vi "4 DDS.vi"(7 "clear DDS":bool, 8 "input valid":bool=TRUE, 9 "pdw in":T2 {"frequency shift" format="%#_12f"}, 10 "free DDS before me?":bool, 11 "new PDW in":bool) -> (0 "output valid":bool, 1 "state of every DDS":bool[](array[boolean]), 2 "have free DDS":bool, 3 "IQ out":T1)   [LabVIEW 2021]
doc: "transmit pulse with one free DDS inside.\nmust have no DDS before him (the distribute is to give the lowest mun DDS the pulse)"
uses:
  pulse_tx_vis/pdw.ctl
  pulse_tx_vis/CTL/mode_type.ctl
  <instrlib>/_niInstr/DSP/v1/Shared/Public/IQ Data.ctl
  <instrlib>/_niInstr/DSP/v1/Shared/niInstr DSP v1 Shared.lvlib
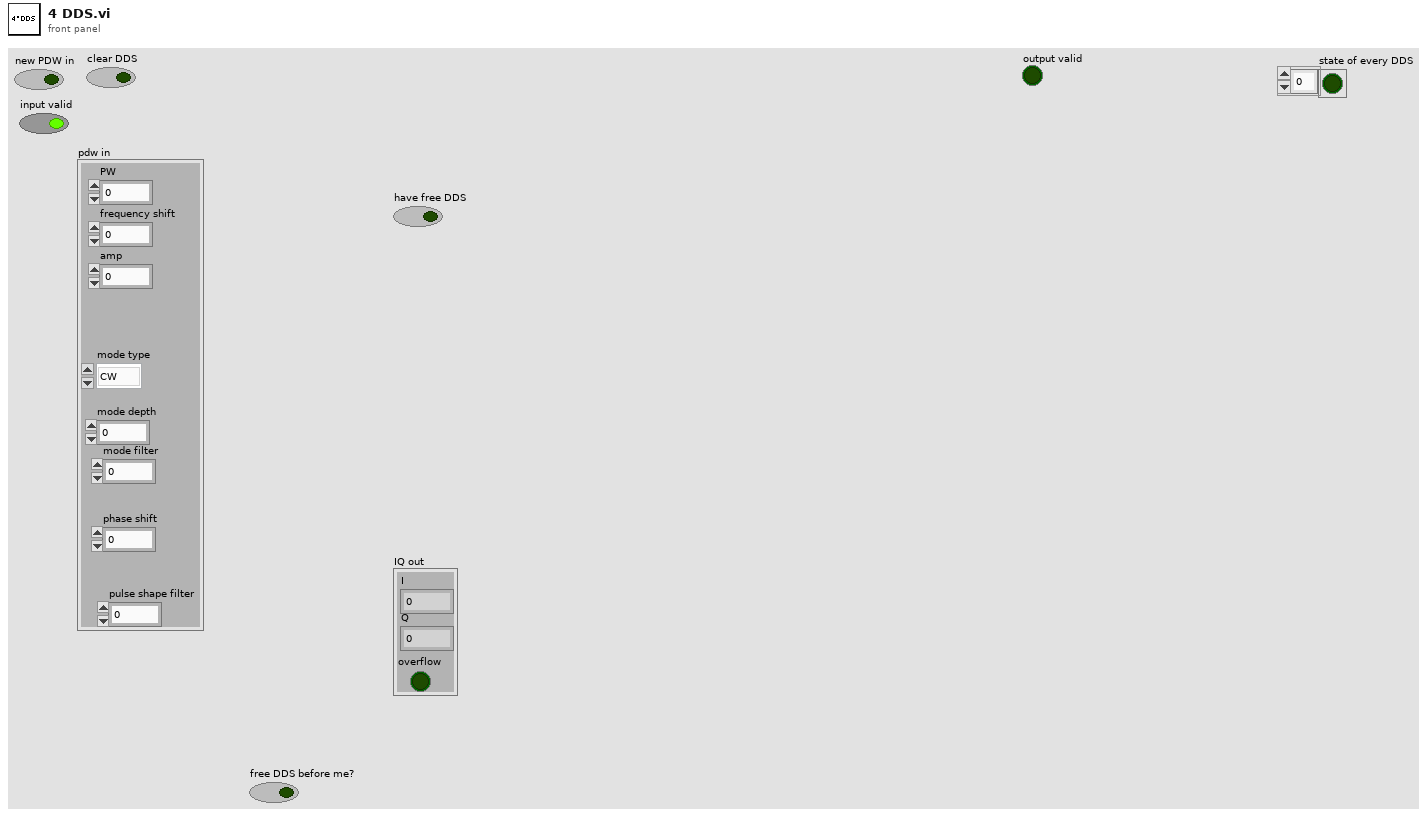
[diagram p1: front panel]
types:
  T1 = typedef "niInstr DSP v1 Shared.lvlib/IQ Data.ctl" = cluster{"I":fxp<+/-,18,1>, "Q":fxp<+/-,18,1>, "overflow":bool}
  T2 = typedef "pdw.ctl" = cluster{"PW":u32, "frequency shift":fxp<+/-,48,0>, "amp":fxp<+/-,18,1>, "mode type":T3, "mode depth":u32, "mode filter":u8, "phase shift":fxp<+/-,16,1>, "pulse shape filter":u8}
  T3 = typedef "mode_type.ctl" = enum8{"CW", "from memory 1", "NC - cw", "LFM", "BPSK", "QPSK"}
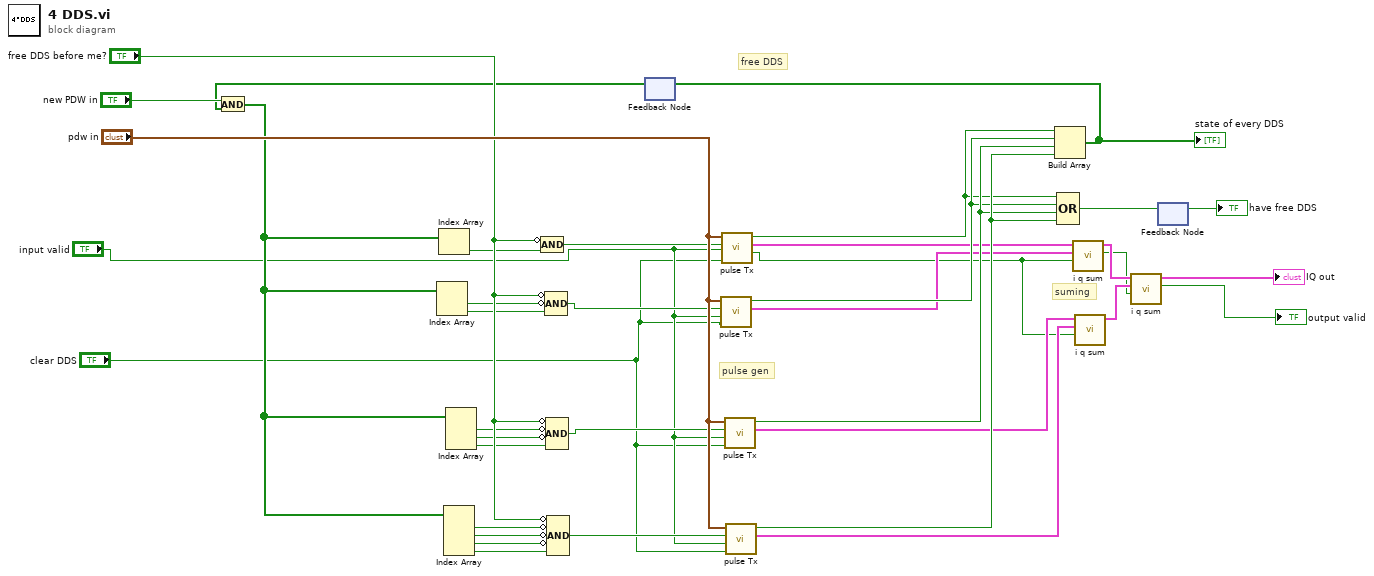
[diagram p0: block diagram]
diagram:
  # "free DDS"
  # "suming"
  # "pulse gen"
  n1 = feedback #1() -> (w9:bool[])  [unwired: 1 in]
  n2 = And(x="new PDW in", y=w9) -> (x .and. y?=w8:bool[])
  n3 = Index Array(array=w8) -> (element #1=w22:bool, element #2=w20:bool)  [unwired: 2 in]
  n4 = Index Array(array=w8) -> (element=w18:bool)  [unwired: 1 in]
  n5 = Index Array(array=w8) -> (element #1=w30:bool, element #2=w29:bool, element #3=w28:bool, element #4=w27:bool)  [unwired: 4 in]
  n6 = Index Array(array=w8) -> (element #1=w26:bool, element #2=w25:bool, element #3=w24:bool)  [unwired: 3 in]
  n7 = Compound Arithmetic op=AND(invert "free DDS before me?", w18) -> (w19:bool)
  n8 = Compound Arithmetic op=AND(invert "free DDS before me?", invert w22, w20) -> (w21:bool)
  n9 = Compound Arithmetic op=AND(invert "free DDS before me?", invert w26, invert w25, w24) -> (w23:bool)
  n10 = Compound Arithmetic op=AND(invert "free DDS before me?", invert w30, invert w29, invert w28, w27) -> (w31:bool)
  n11 = call "pulse Tx.vi"("clear DDS"="clear DDS", "enable line"="input valid", "take it!"=w21, "Cluster"="pdw in") -> ("data out"=w15:T1, "free dds"=w34:bool)  [unwired: 3 in, 3 out]
  n12 = call "pulse Tx.vi"("clear DDS"="clear DDS", "enable line"="input valid", "take it!"=w19, "Cluster"="pdw in") -> ("output valid"=w4:bool, "data out"=w14:T1, "free dds"=w33:bool)  [unwired: 3 in, 2 out]
  n13 = call "pulse Tx.vi"("clear DDS"="clear DDS", "enable line"="input valid", "take it!"=w23, "Cluster"="pdw in") -> ("data out"=w16:T1, "free dds"=w35:bool)  [unwired: 3 in, 3 out]
  n14 = call "pulse Tx.vi"("clear DDS"="clear DDS", "enable line"="input valid", "take it!"=w31, "Cluster"="pdw in") -> ("data out"=w17:T1, "free dds"=w36:bool)  [unwired: 3 in, 3 out]
  n15 = Build Array(w33, w34, w35, w36) -> (w11:bool[])
  "state of every DDS" <- w11
  n16 = feedback-in #1(w11) -> ()
  n17 = Compound Arithmetic op=OR(w33, w34, w35, w36) -> (w7:bool)
  n18 = call "i q sum.vi"("input valid"=w4, 10:"data in"=w15, 11:"data in"=w14) -> ("output valid"=w3:bool, "output cluster"=w13:T1)  [unwired: 7 in]
  n19 = call "i q sum.vi"("input valid"=w4, 10:"data in"=w17, 11:"data in"=w16) -> ("output cluster"=w12:T1)  [unwired: 7 in, 1 out]
  n20 = call "i q sum.vi"("input valid"=w3, 10:"data in"=w12, 11:"data in"=w13) -> ("output valid"=→"output valid":bool, "output cluster"=→"IQ out":T1)  [unwired: 7 in]
  n21 = feedback #2() -> (→"have free DDS":bool)  [unwired: 1 in]
  n22 = feedback-in #2(w7) -> ()
